vi "Sync clock to NIST time.vi"(10 "Time zone selector":string="America/New_York", 11 "NIST time server IP address":string="time.nist.gov") -> (3 "Sync OK":bool)   [LabVIEW 2021]
uses:
  <vilib>/Utility/miscctls.llb/LVDateTimeRec.ctl
  <vilib>/nisyscfg/nisyscfg.lvlib
panel:
  out "returned ITS string":string
  out "error out":errorcluster
  in  "error in (no error)":errorcluster
  in  "Century Number":i32=21
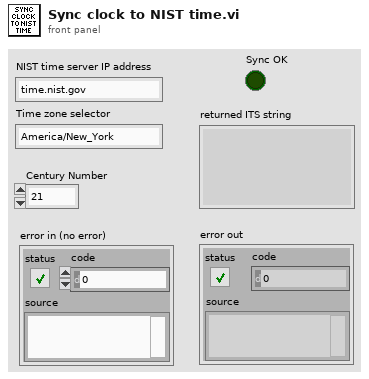
[diagram p1: front panel]
types:
  T1 = typedef "LVDateTimeRec.ctl" = cluster{"fractional second":dbl, "second":i32, "minute":i32, "hour":i32, "day of month":i32, "month":i32, "year":i32, "day of week":i32, "day of year":i32, "DST":i32}
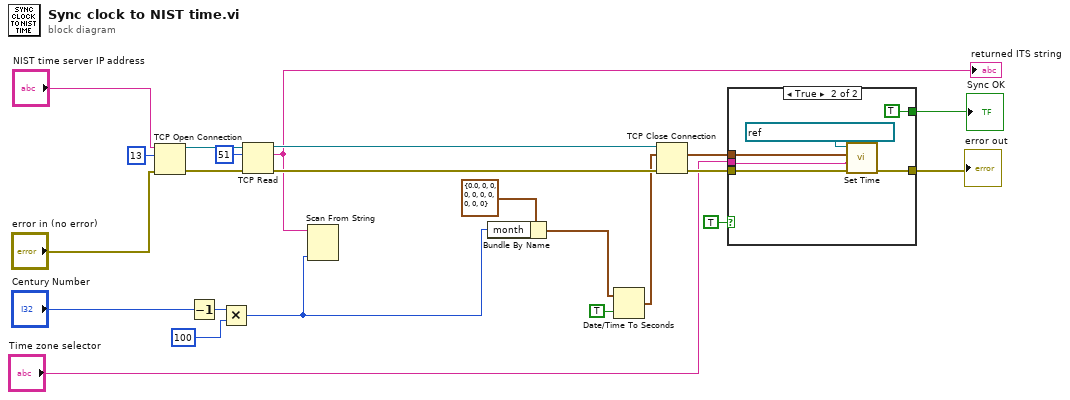
[diagram p0: block diagram]
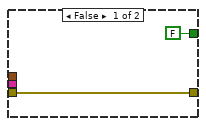
[diagram p2: hidden frame]
diagram:
  n1 = TCP Open Connection(address="NIST time server IP address", remote port or service name=u16 13, error in (no error)="error in (no error)") -> (connection ID=w15:refnum<k5>, error out=w19:errorcluster)  [unwired: 2 in]
  n2 = Decrement(x="Century Number") -> (x-1=w6:i32)
  n3 = Multiply(x=w6, y=100) -> (x*y=w2:i32)
  n4 = TCP Read(connection ID=w15, bytes to read=51, error in (no error)=w19) -> (connection ID out=w14:refnum<k5>, data out=w8:string, error out=w20:errorcluster)  [unwired: 2 in]
  "returned ITS string" <- w8
  n5 = Scan From String(input string=w8, default 1=w2) -> ()  [unwired: 4 in, 3 out]
  n6 = Bundle By Name(cluster=T1 {"fractional second"=0.0, "second"=0, "minute"=0, "hour"=0, "day of month"=0, "month"=0, "year"=0, "day of week"=0, "day of year"=0, "DST"=0} ("date time rec"), "month"=w2) -> (w3:T1)
  n7 = Date/Time To Seconds(1:TRUE ("is UTC (F)"), 2:w3) -> (0:w9:timestamp)
  n8 = TCP Close Connection(connection ID=w14, error in (no error)=w20) -> (error out=w21:errorcluster)  [unwired: 1 in, 1 out]
  n9 = case shown="True" TRUE {
    tunnel: [w24 w29] -> w22
    tunnel: w21 -> [w24 w28]
    tunnel: "Time zone selector" -> [_ w27]
    tunnel: [FALSE ("Sync OK") TRUE ("Sync OK")] -> w11
    tunnel: w9 -> [_ w25]
    frame False {
    }
    frame True {
      n10 = call <vilib>:"Set Time.vi"("error in (no error)"=w28, "Time Zone"=w27, "Time"=w25, "Session in (localhost)"=refnum<k21> "myRIO-1900 (10.0.0.46)") -> ("error out"=w29:errorcluster)  [unwired: 4 in, 3 out]
    }
  }
  "Sync OK" <- w11
  "error out" <- w22
